vi "merge.vi"(8 "error in (no error)":errorcluster, 9 "all?":bool, 10 "bunch size":i32=1 min=1, 11 "ImageCollection in":refnum<class "ImageCollection.lvclass">) -> (0 "error out":errorcluster, 3 "ImageCollection out":refnum<class "ImageCollection.lvclass">)   [LabVIEW 2010, in "ImageCollection.lvclass"]
uses:
  ImageCollection.lvclass
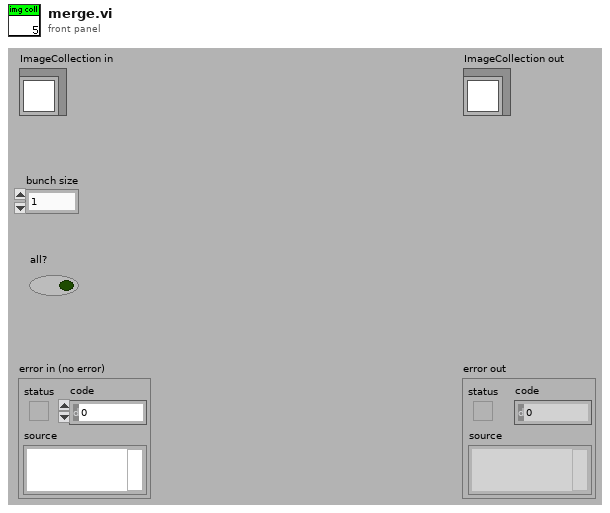
[diagram p1: front panel]
types:
  T1 = typedef "ImageCollection.lvclass/storage_mode_enum.ctl" = enum16{"RAM", "single files", "multipage TIFF (read-only)"}
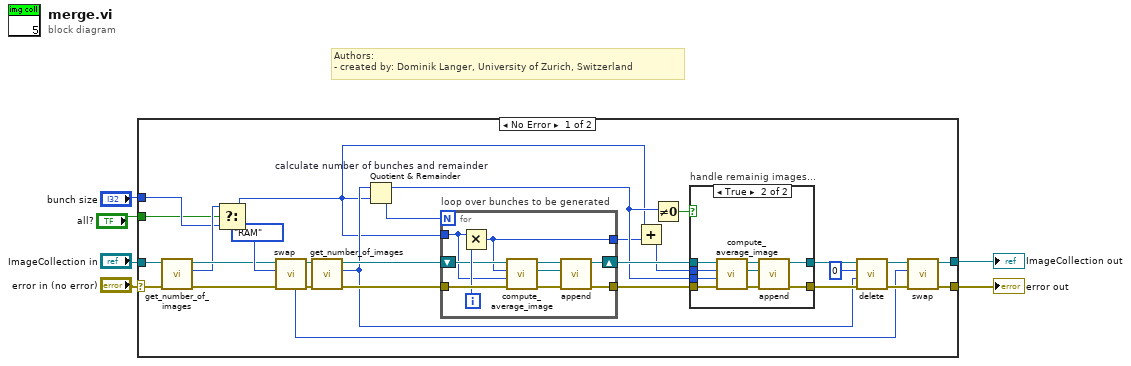
[diagram p0: block diagram]
diagram:
  # "Authors: \n- created by: Dominik Langer, University of Zurich, Switzerland"
  n1 = case shown="No Error" "error in (no error)" {
    selector: "error in (no error)" -> [w14 w57]
    tunnel: [w30 w57] -> w5
    tunnel: [w28 w56] -> w3
    tunnel: "ImageCollection in" -> [w13 w56]
    tunnel: "bunch size" -> [w9 _]
    tunnel: "all?" -> [w7 _]
    frame No Error {
      n2 = call-dynamic "get_number_of_images.vi"("error in (no error)"=w14, "ImageCollection in"=w13) -> ("error out"=w12:errorcluster, "size"=w10:i32, "ImageCollection out"=w11:refnum<class "ImageCollection.lvclass">)  [unwired: 7 out]
      n3 = Select(t=w10, s=w7, f=w9) -> (s? t:f=w8:i32)
      n4 = call-dynamic "swap.vi"("error in (no error)"=w12, "target storage mode"=enum16{"RAM", "single files"}."RAM", "ImageCollection in"=w11) -> ("error out"=w33:errorcluster, "ImageCollection out"=w34:refnum<class "ImageCollection.lvclass">, "previous storage mode"=w27:T1)  [unwired: 6 out]
      n5 = call-dynamic "get_number_of_images.vi"("error in (no error)"=w33, "ImageCollection in"=w34) -> ("error out"=w25:errorcluster, "size"=w21:i32)  [unwired: 8 out]
      n6 = Quotient & Remainder "calculate number of bunches and remainder"(x=w21, y=w8) -> (x-y*floor(x/y)=w17:i32, floor(x/y)=w20:i32)
      n7 = for "loop over bunches to be generated" {
        N: w20 -> [_]
        tunnel: w25 -> [w55]
        tunnel: w8 -> [w46]
        tunnel: [w51] -> w26
        shift-right: [w50] -> w22
        shift-left: w34 -> [w49]
        tunnel: [w47] -> w16
        i -> [w54]
        n8 = Multiply(x=w46, y=w54) -> (x*y=w47:i32)
        n9 = call-dynamic "compute_average_image.vi"("error in (no error)"=w55, "range"=w46, "start index"=w47, "ImageCollection in"=w49) -> ("error out"=w52:errorcluster, "averaged image"=w53:refnum<class "Image.lvclass">, "ImageCollection out"=w48:refnum<class "ImageCollection.lvclass">)  [unwired: 1 in, 4 out]
        n10 = call-dynamic "append.vi"("error in (no error)"=w52, "Image.lvclass"=w53, "ImageCollection in"=w48) -> ("error out"=w51:errorcluster, "ImageCollection out"=w50:refnum<class "ImageCollection.lvclass">)  [unwired: 1 in, 6 out]
      }
      n11 = Add(x=w8, y=w16) -> (x+y=w15:i32)
      n12 = Not Equal To 0?(x=w17) -> (x != 0?=w18:bool)
      n13 = case "handle remainig images..." shown="True" w18 {
        tunnel: w26 -> [w36 w43]
        tunnel: w15 -> [_ w42]
        tunnel: [w36 w41] -> w24
        tunnel: [w35 w40] -> w23
        tunnel: w22 -> [w35 w39]
        tunnel: w17 -> [_ w37]
        frame False {
        }
        frame True {
          n14 = call-dynamic "compute_average_image.vi"("error in (no error)"=w43, "range"=w37, "start index"=w42, "ImageCollection in"=w39) -> ("error out"=w44:errorcluster, "averaged image"=w45:refnum<class "Image.lvclass">, "ImageCollection out"=w38:refnum<class "ImageCollection.lvclass">)  [unwired: 1 in, 4 out]
          n15 = call-dynamic "append.vi"("error in (no error)"=w44, "Image.lvclass"=w45, "ImageCollection in"=w38) -> ("error out"=w41:errorcluster, "ImageCollection out"=w40:refnum<class "ImageCollection.lvclass">)  [unwired: 1 in, 6 out]
        }
      }
      n16 = call-dynamic "delete.vi"("error in (no error)"=w24, "range"=w21, "start index"=0, "ImageCollection in"=w23) -> ("error out"=w31:errorcluster, "ImageCollection out"=w29:refnum<class "ImageCollection.lvclass">)  [unwired: 6 out]
      n17 = call-dynamic "swap.vi"("error in (no error)"=w31, "target storage mode"=w27, "ImageCollection in"=w29) -> ("error out"=w30:errorcluster, "ImageCollection out"=w28:refnum<class "ImageCollection.lvclass">)  [unwired: 7 out]
    }
    frame Error {
    }
  }
  "error out" <- w5
  "ImageCollection out" <- w3
